vi "BadRequestError.vi"(11 "JQMHModule in":refnum<class "RQMHModule.lvclass">) -> (0 "error out":errorcluster, 3 "JQMHModule out":refnum<class "RQMHModule.lvclass">)   [LabVIEW 2024, in "RQMHModule.lvclass"]
uses:
  RQMHModule.lvclass
  RQMHModule.lvclass/RQMHModule.ctl
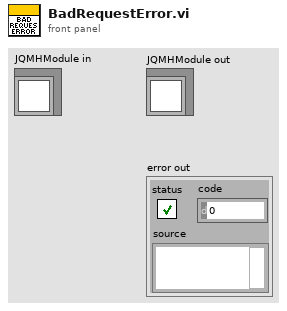
[diagram p1: front panel]
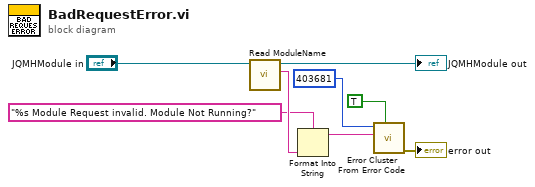
[diagram p0: block diagram]
diagram:
  n1 = call "Read ModuleName.vi"("JQMHModule in"="JQMHModule in") -> ("ModuleName"=w7:string, "JQMHModule out"=→"JQMHModule out":refnum<class "RQMHModule.lvclass">)  [unwired: 8 in, 1 out]
  n2 = Format Into String(format string="%s Module Request invalid. Module Not Running?" ("error message (\"\")"), w7) -> (resulting string=w6:string)  [unwired: 2 in, 1 out]
  n3 = call <vilib>:"Error Cluster From Error Code.vi"("show call chain? (False)"=TRUE, "error message (\"\")"=w6, "error code (0)"=403681) -> ("error out"=→"error out":errorcluster)  [unwired: 6 in]
